vi "CH_LM Calibration Calibrate Output.vi"(0 "Meter Index":i32, 2 "Counts at 0V":i32, 3 "Counts at 4V":i32, 5 "error in (no error)":errorcluster, 7 "Timeout / ms (3000)":i32=3000, 9 "Lock Timeout / ms (1000)":i32=1000) -> (11 "Lock timed out":bool, 14 "Meter Index":i32, 19 "error out":errorcluster)   [LabVIEW 2012, in "CH_LM.lvlib"]
doc: "This command calibrates the analog output voltage.\n\n<B>Counts at 0V</B> and <B>Counts at 5V</B> are calculated values and, hence, might sometimes range beyond the capability of the DAC."
uses:
  CH_LM.lvlib
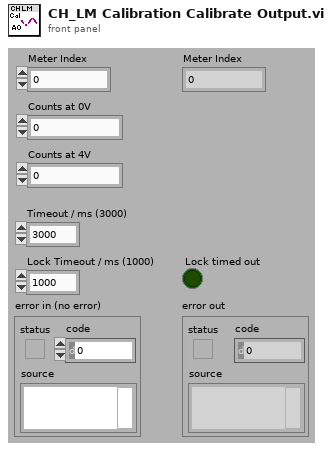
[diagram p1: front panel]
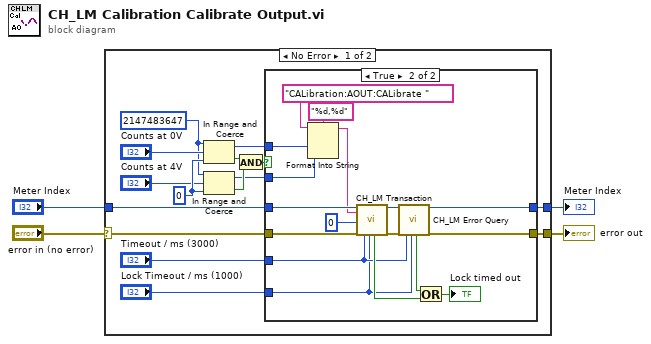
[diagram p0: block diagram]
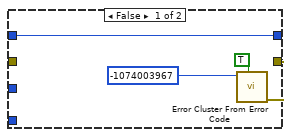
[diagram p2: hidden frame]
diagram:
  n1 = case shown="No Error" "error in (no error)" {
    selector: "error in (no error)" -> [w19 w42]
    tunnel: [w16 w42] -> w4
    tunnel: "Meter Index" -> [w18 w41]
    tunnel: [w17 w41] -> w1
    frame No Error {
      w6 = 2147483647 ("upper limit")
      w7 = 0 ("lower limit")
      n2 = In Range and Coerce(upper limit=w6, x="Counts at 0V", lower limit=w7) -> (coerced(x)=w12:i32, In Range?=w10:bool)
      n3 = In Range and Coerce(upper limit=w6, x="Counts at 4V", lower limit=w7) -> (coerced(x)=w8:i32, In Range?=w11:bool)
      n4 = And(x=w10, y=w11) -> (x .and. y?=w9:bool)
      n5 = case shown="True" w9 {
        tunnel: w19 -> [_ w40]
        tunnel: w18 -> [w23 w39]
        tunnel: [w23 w38] -> w17
        tunnel: [w20 w37] -> w16
        tunnel: "Timeout / ms (3000)" -> [_ w33]
        tunnel: "Lock Timeout / ms (1000)" -> [_ w32]
        tunnel: w12 -> [_ w31]
        tunnel: w8 -> [_ w28]
        frame False {
          n6 = call <vilib>:"Error Cluster From Error Code.vi"("show call chain? (False)"=TRUE, "error code (0)"=-1074003967) -> ("error out"=w20:errorcluster)  [unwired: 1 in, 6 out]
        }
        frame True {
          n7 = Format Into String(format string="%d,%d", initial string="CALibration:AOUT:CALibrate ", w31, w28) -> (resulting string=w29:string)  [unwired: 1 in, 1 out]
          n8 = call "CH_LM Transaction.vi"("Meter Index"=w39, "Command String"=w29, "NofStrings (-1:all)"=0, "error in (no error)"=w40, "Timeout / ms (3000)"=w33, "Lock Timeout / ms (1000)"=w32) -> ("Lock timed out"=w35:bool, "Meter Index"=w26:i32, "error out"=w25:errorcluster)  [unwired: 11 out]
          n9 = call "CH_LM Error Query.vi"("Meter Index"=w26, "error in (no error)"=w25, "Timeout / ms (3000)"=w33, "Lock Timeout / ms (1000)"=w32) -> ("Lock timed out"=w36:bool, "Meter Index"=w38:i32, "error out"=w37:errorcluster)  [unwired: 13 out]
          n10 = Or(x=w36, y=w35) -> (x .or. y?=→"Lock timed out":bool)
        }
      }
    }
    frame Error {
    }
  }
  "error out" <- w4
  "Meter Index" <- w1
